vi "Read Acceleration.vi"(8 "error in (no error)":errorcluster, 11 "Motion Controller in":refnum<class "Motion Controller.lvclass">) -> (0 "error out":errorcluster, 2 "Acceleration":dbl[](array[numeric]), 3 "Motion Controller out":refnum<class "Motion Controller.lvclass">)   [LabVIEW 2022 SP3, in "Motion Controller.lvclass"]
uses:
  Motion Controller.lvclass
  Motion Controller.lvclass/Motion Controller.ctl
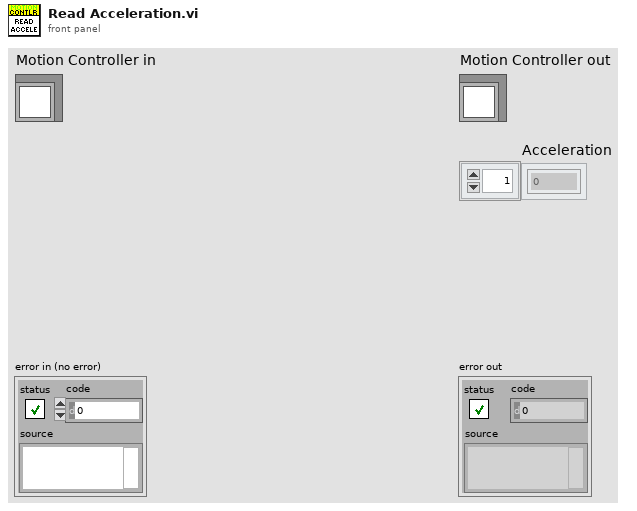
[diagram p1: front panel]
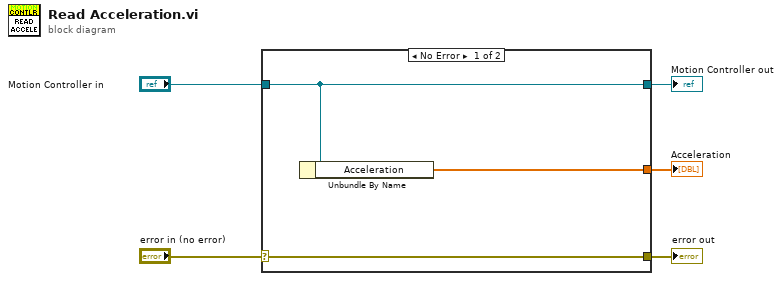
[diagram p0: block diagram]
diagram:
  n1 = case shown="No Error" "error in (no error)" {
    selector: "error in (no error)" -> [w8 w9]
    tunnel: [w8 w9] -> w4
    tunnel: [w7 w10] -> w2
    tunnel: "Motion Controller in" -> [w7 w10]
    tunnel: [w6 _] -> w1
    frame No Error {
      n2 = Unbundle By Name(w7) -> ("Acceleration"=w6:dbl[])
    }
    frame Error {
    }
  }
  "error out" <- w4
  "Motion Controller out" <- w2
  "Acceleration" <- w1
